vi "sequence_edited.vi"() -> ()   [LabVIEW 2020]
uses:
  C:/Users/Public/Documents/Photometrics/PMQI-LabViewSamples/Examples/2018/Dependencies/PVCamNET.dll
  Dependencies/PVCamNET.dll
panel:
  in  "Path":path
  out "SavingPath":string
  out "Boolean":bool
  in  "?":bool
  out "Capturing":bool
  in  "?":bool
  in  "FramesToCapture":u16
  in  "Exposure":u32
  in  "?":bool
  # "Description:\nThis code lets the user use sequence mode and save a TIFF image with \nthe user's preferred buffer size (framesToCapture) and exposure time. \n\nSteps to run:\n1. Update Path (Example: d:\\Temp\\ )\n2. Click \"Run\"\n3. Enter FramesToCapture and Exposure time\n4. Click \"START\"\n5. Click \"SAVE\"\n6. Click \"CLOSE\""
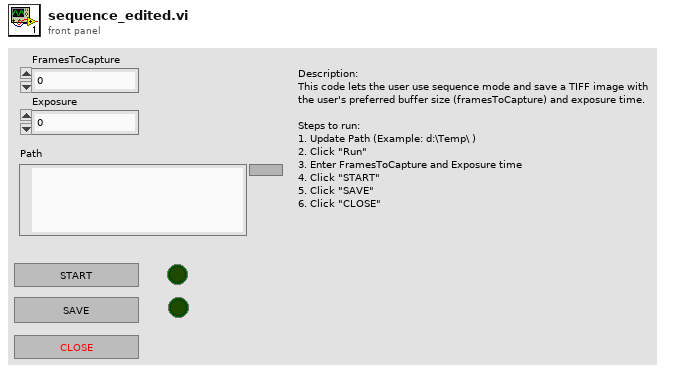
[diagram p1: front panel]
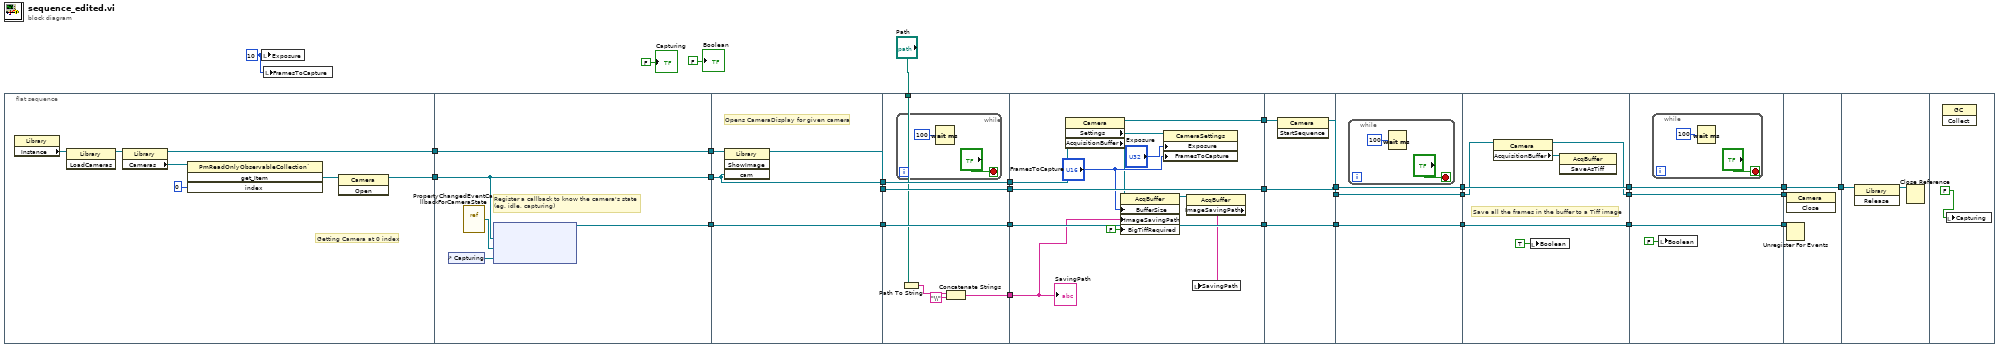
[diagram p0: block diagram]
diagram:
  w13 = u32 10 ("Exposure")
  n1 = flat-sequence {
    tunnel: [w35] -> w32
    tunnel: [w36] -> w31
    tunnel: w32 -> [w44]
    tunnel: [w44] -> w30
    tunnel: w31 -> [w41]
    tunnel: [w41] -> w29
    tunnel: [w40] -> w28
    tunnel: w30 -> [w48]
    tunnel: w29 -> [w47]
    tunnel: [w47] -> w26
    tunnel: [w46] -> w27
    tunnel: [w45] -> w25
    tunnel: w28 -> [w45]
    tunnel: w27 -> [w55]
    tunnel: [w55] -> w24
    tunnel: w26 -> [w54]
    tunnel: [w54] -> w23
    tunnel: [w53] -> w22
    tunnel: w25 -> [w53]
    tunnel: [w50] -> w2
    tunnel: "Path" -> [w49]
    tunnel: [w69] -> w21
    tunnel: [w68] -> w20
    tunnel: w24 -> [w68]
    tunnel: w23 -> [w67]
    tunnel: [w64] -> w19
    tunnel: w22 -> [w64]
    tunnel: w2 -> [w58]
    tunnel: w21 -> [w71]
    tunnel: [w70] -> w18
    tunnel: w20 -> [w73]
    tunnel: [w73] -> w17
    tunnel: [w72] -> w16
    tunnel: w19 -> [w72]
    tunnel: w18 -> [w76]
    tunnel: [w76] -> w12
    tunnel: w17 -> [w75]
    tunnel: [w75] -> w11
    tunnel: w16 -> [w74]
    tunnel: [w74] -> w10
    tunnel: w12 -> [w81]
    tunnel: [w80] -> w9
    tunnel: w11 -> [w84]
    tunnel: [w84] -> w7
    tunnel: w10 -> [w83]
    tunnel: [w83] -> w5
    tunnel: w9 -> [w88]
    tunnel: [w88] -> w8
    tunnel: w7 -> [w87]
    tunnel: [w87] -> w6
    tunnel: w5 -> [w86]
    tunnel: [w86] -> w4
    tunnel: w8 -> [w93]
    tunnel: w6 -> [w92]
    tunnel: [w92] -> w15
    tunnel: w4 -> [w91]
    tunnel: w15 -> [w95]
    frame #0 {
      # "Getting Camera at 0 index"
      n2 = property class="Library"() -> ("Instance"=w34:refnum<k24>)  [unwired: 2 in, 2 out]
      n3 = invoke class="Library" method="LoadCameras"(reference=w34) -> (reference out=w33:refnum<k24>)  [unwired: 2 in, 2 out]
      n4 = property class="Library"(reference=w33) -> (reference out=w35:refnum<k24>, "Cameras"=w39:refnum<k24>)  [unwired: 1 in, 1 out]
      n5 = invoke class="PmReadOnlyObservableCollection`" method="get_Item"(reference=w39, "index"=0) -> ("get_Item"=w37:refnum<k24>)  [unwired: 2 in, 3 out]
      n6 = invoke class="Camera" method="Open"(reference=w37) -> (reference out=w36:refnum<k24>)  [unwired: 2 in, 2 out]
    }
    frame #1 {
      # "Register a callback to know the camera's state \n(eg. idle, capturing)"
      n7 = control-ref of="Capturing"() -> (w43:refnum<vi>)
      n8 = vi-ref "PropertyChangedEventCallbackForCameraState.vi"() -> ("vi reference"=w42:refnum<vi>)
      n9 = node(w41, w42, w43) -> (w40:refnum<k27>)  [unwired: 2 in, 1 out]
    }
    frame #2 {
      # "Opens CameraDisplay for given camera"
      n10 = invoke class="Library" method="ShowImage"(reference=w48, "cam"=w47) -> (reference out=w46:refnum<k24>)  [unwired: 2 in, 3 out]
    }
    frame #3 {
      n11 = while {
        stop <- "?" stop-if-true
        n12 = Wait (ms)(milliseconds to wait=u32 100) -> ()  [unwired: 1 out]
      }
      n13 = Path To String(path=w49) -> (string=w52:string)
      n14 = Concatenate Strings(w52, "\\" ("string")) -> (w50:string)
    }
    frame #4 {
      n15 = property class="Camera"(reference=w67) -> (reference out=w69:refnum<k24>, "Settings"=w66:refnum<k24>, "AcquisitionBuffer"=w62:refnum<k24>)  [unwired: 1 in, 1 out]
      n16 = property class="AcqBuffer"(reference=w62, "BufferSize"="FramesToCapture", "ImageSavingPath"=w58, "BigTiffRequired"=FALSE) -> (reference out=w61:refnum<k24>)  [unwired: 1 in, 1 out]
      n17 = property class="CameraSettings"(reference=w66, "Exposure"="Exposure", "FramesToCapture"="FramesToCapture") -> ()  [unwired: 1 in, 2 out]
      n18 = property class="AcqBuffer"(reference=w61) -> ("ImageSavingPath"=w59:string)  [unwired: 1 in, 2 out]
      n19 = local write "SavingPath"(w59) -> ()
      "SavingPath" <- w58
    }
    frame #5 {
      n20 = invoke class="Camera" method="StartSequence"(reference=w71) -> (reference out=w70:refnum<k24>)  [unwired: 2 in, 2 out]
    }
    frame #6 {
      n21 = while {
        stop <- "?" stop-if-true
        n22 = Wait (ms)(milliseconds to wait=u32 100) -> ()  [unwired: 1 out]
      }
    }
    frame #7 {
      # "Save all the frames in the buffer to a Tiff image"
      n23 = property class="Camera"(reference=w81) -> (reference out=w80:refnum<k24>, "AcquisitionBuffer"=w82:refnum<k24>)  [unwired: 1 in, 1 out]
      n24 = local write "Boolean"(TRUE ("Boolean")) -> ()
      n25 = invoke class="AcqBuffer" method="SaveAsTiff"(reference=w82) -> ()  [unwired: 2 in, 3 out]
    }
    frame #8 {
      n26 = while {
        stop <- "?" stop-if-true
        n27 = Wait (ms)(milliseconds to wait=u32 100) -> ()  [unwired: 1 out]
      }
      n28 = local write "Boolean"(FALSE ("Boolean")) -> ()
    }
    frame #9 {
      n29 = invoke class="Camera" method="Close"(reference=w93) -> ()  [unwired: 2 in, 3 out]
      n30 = Unregister For Events(event registration refnum=w91) -> ()  [unwired: 1 in, 1 out]
    }
    frame #10 {
      n31 = invoke class="Library" method="Release"(reference=w95) -> (reference out=w94:refnum<k24>)  [unwired: 2 in, 2 out]
      n32 = Close Reference(reference=w94) -> ()  [unwired: 1 in, 1 out]
    }
    frame #11 {
      n33 = invoke class="GC" method="Collect"() -> ()  [unwired: 3 in, 3 out]
      n34 = local write "Capturing"(FALSE ("Boolean")) -> ()
    }
  }
  n35 = local write "Exposure"(w13) -> ()
  n36 = local write "FramesToCapture"(w13) -> ()
  "Capturing" <- FALSE ("Capturing")
  "Boolean" <- FALSE ("Boolean")
